vi "datascope.to_json.vi"(8 "error in":errorcluster, 10 "data scope":T1) -> (0 "error out":errorcluster, 2 "json":string)   [LabVIEW 2020, in "dataScopes.lvlib"]
uses:
  dataScopes.lvlib
  data_scope.ctl
  data_source.ctl
  type.ctl
  offset.ctl
  b3ef6cc6-145b-425d-8ca9-b3251dbecc9c.vi
  <vilib>/JDP Science/JSONtext/Variant to JSON Text.vi
  <vilib>/JDP Science/JSONtext/support/Format JSON Object.vi
  <vilib>/JDP Science/JSONtext/LVClass Serializer/JSONtext LVClass Serializer.lvclass
  properties/properties.lvclass
  <vilib>/JDP Science/JSONtext/JSONtext.lvlib
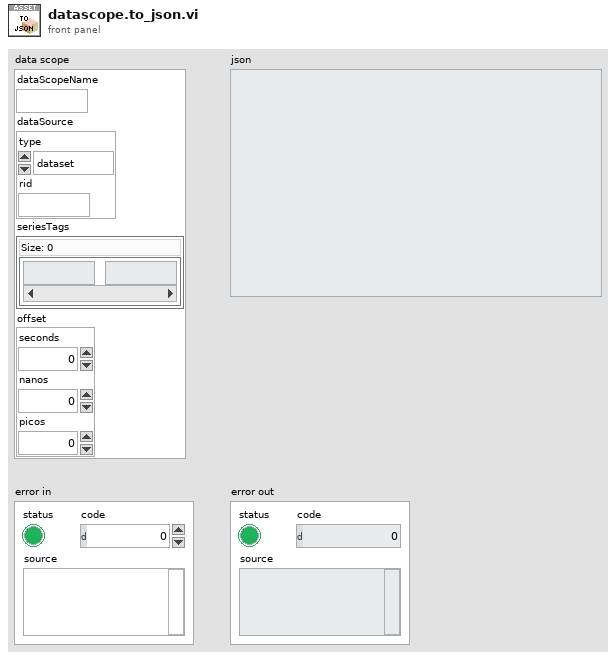
[diagram p1: front panel]
types:
  T1 = typedef "dataScopes.lvlib/data_scope.ctl" = cluster{"dataScopeName":string, "dataSource":T2, "seriesTags":map{string, string}, "offset":T4}
  T2 = typedef "dataScopes.lvlib/data_source.ctl" = cluster{"type":T3, "rid":string}
  T3 = typedef "dataScopes.lvlib/type.ctl" = enum16{"dataset", "connection", "logSet", "video"}
  T4 = typedef "dataScopes.lvlib/offset.ctl" = cluster{"seconds":i32, "nanos":i32, "picos":i32}
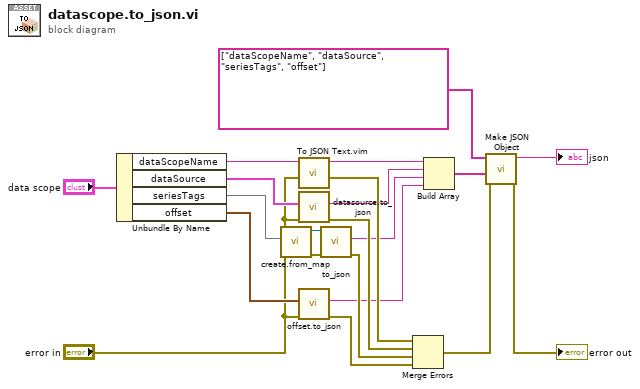
[diagram p0: block diagram]
diagram:
  n1 = Unbundle By Name("data scope") -> ("dataScopeName"=w20:string, "dataSource"=w9:T2, "seriesTags"=w4:map{string, string}, "offset"=w8:T4)
  n2 = call "create.from_map.vi"("error in"="error in", "properties"=w4) -> ("error out"=w2:errorcluster, "properties out"=w3:refnum<class "properties.lvclass">)  [unwired: 8 in]
  n3 = call "To JSON Text.vim"("error in (no error)"="error in", "Anything"=w20) -> ("error out"=w15:errorcluster, "<JSON>"=w19:string)  [unwired: 8 in]
  n4 = call "datasource.to_json.vi"("error in"="error in", "dataSource"=w9) -> ("error out"=w14:errorcluster, "json"=w7:string)  [unwired: 8 in]
  n5 = call "offset.to_json.vi"("error in"="error in", "offset"=w8) -> ("error out"=w12:errorcluster, "json"=w6:string)  [unwired: 8 in]
  n6 = call-dynamic "to_json.vi"("error in"=w2, "properties in"=w3) -> ("error out"=w13:errorcluster, "json"=w5:string)  [unwired: 6 in, 2 out]
  n7 = Merge Errors(w15, w14, w13, w12) -> (w11:errorcluster)
  n8 = Build Array(w19, w7, w5, w6) -> (w18:string[])
  n9 = call <vilib>:"Make JSON Object.vi"("error in (no error)"=w11, "JSON Items"=w18, "Item Names"=string[] ["dataScopeName", "dataSource", "seriesTags", "offset"]) -> ("error out"=→"error out":errorcluster, "<JSON>"=→"json":string)  [unwired: 7 in]
